vi "Check Debug.vi"(8 "error in (no error)":errorcluster, 11 "Volatus Core in":refnum<class "Volatus Core.lvclass">) -> (0 "error out":errorcluster, 3 "Volatus Core out":refnum<class "Volatus Core.lvclass">)   [LabVIEW 2020, in "Volatus.lvlib" / "Volatus Core.lvclass"]
uses:
  Volatus Core.lvclass
  Volatus Core.lvclass/Volatus Core.ctl
  Module/Module.lvclass
  lv-cdm/CDM-Config/Config Element/Config Element.lvclass
  C:/dev/lv20CE/relink/lv-volatus/Volatus/Module/Module.lvclass
  C:/dev/lv20CE/relink/lv-volatus/Volatus/Volatus Core/Volatus Core.lvclass
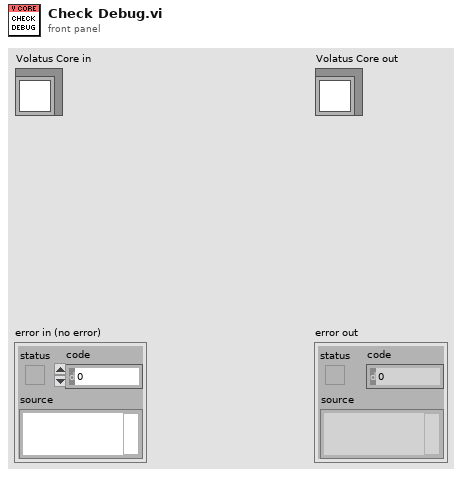
[diagram p1: front panel]
types:
  T1 = enum32{"invalid app kind", "Development System", "Run Time System", "Student Edition", "Embedded LabVIEW", "Evaluation", "Custom"}
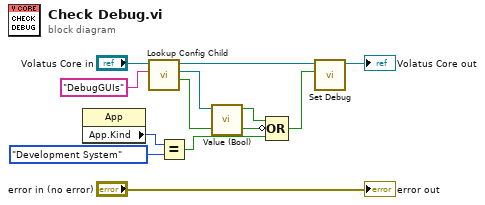
[diagram p0: block diagram]
diagram:
  n1 = property class="App"() -> ("App.Kind"=w10:T1)  [unwired: 2 in, 2 out]
  n2 = call "Lookup Config Child.vi"("Name"="DebugGUIs", "Module in"="Volatus Core in") -> ("Found"=w4:bool, "Config Child"=w6:refnum<class "Config Element.lvclass">, "Module out"=w8:refnum<class "Volatus Core.lvclass">)  [unwired: 6 in, 1 out]
  n3 = Equal?(x=w10, y=T1."Development System") -> (x = y?=w3:bool)
  n4 = call "Value (Bool).vi"("Config Element in"=w6) -> ("Bool Value"=w5:bool)  [unwired: 9 in, 1 out]
  n5 = Compound Arithmetic op=OR(w5, invert w4, w3) -> (w1:bool)
  n6 = call "Set Debug.vi"("Debug"=w1, "Module in"=w8) -> ("Module out"=→"Volatus Core out":refnum<class "Volatus Core.lvclass">)  [unwired: 9 in]
  "error out" <- "error in (no error)"
